vi "SingleAxis_MoveInc_MoveAbs_Home.vi"() -> ()   [LabVIEW 2016]
uses:
  Examples/Motion/EnableSingle.vi
  Examples/Motion/MoveIncSingle.vi
  Examples/Motion/WaitSingle.vi
  Examples/Motion/MoveAbsSingle.vi
  Examples/Motion/HomeSingle.vi
  Examples/Motion/DisableSingle.vi
panel:
  out "FinalPosition":string
  in  "MoveAbsPosition":dbl
  in  "MoveAbsSpeed":dbl
  in  "MoveIncDistance":dbl
  in  "MoveIncSpeed":dbl
  in  "AxisName":string
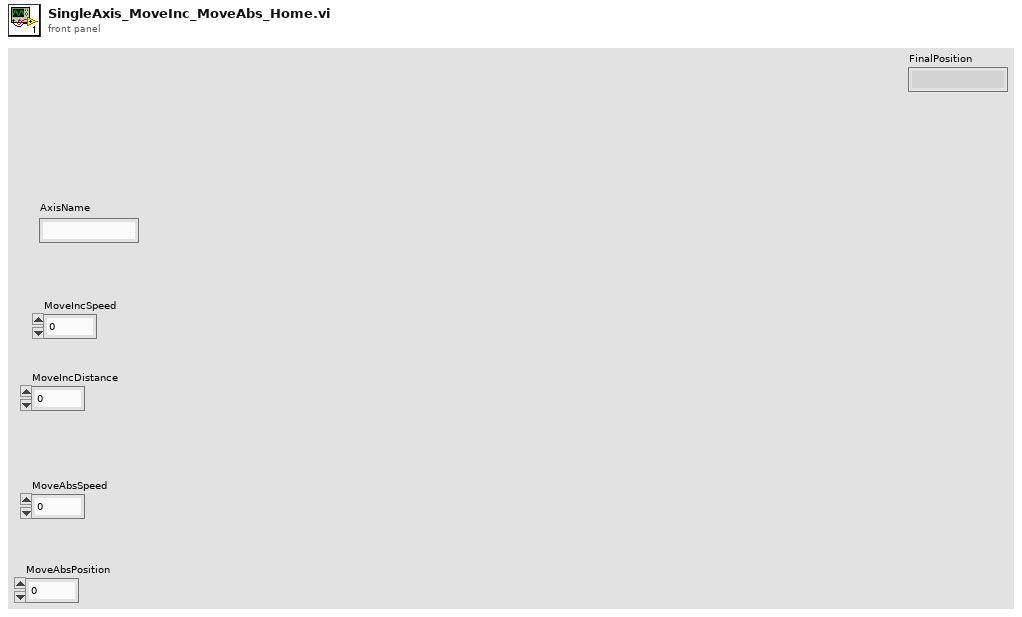
[diagram p1: front panel]
types:
  T1 = typedef "ControllerDiagPacket.ctl" = cluster{"Number of Diag Packets":i32, "Axes":T2[], "error":errorcluster}
  T2 = typedef "AxisDiagPacket.ctl" = cluster{"Axis Name":string, "Analog Input 0":dbl, "Analog Input 1":dbl, "Axis Fault (num)":i32, "Axis Fault (str)":string, "Axis Fault (bits)":cluster{"AmplifierFault":bool, "AmplifierTemperatureFault":bool, "CcwEndOfTravelLimitFault":bool, "CcwSoftwareLimitFault":bool, "CommunicationLostFault":bool, "CwEndOfTravelLimitFault":bool, "CwSoftwareLimitFault":bool, "EmergencyStopFault":bool, "EncoderFault":bool, "ExternalFault":bool, "FeedbackScalingFault":bool, "GantryMisalignFault ":bool, "HallSensorFault":bool, "InPositionTimeoutFault":bool, "MarkerSearchFault":bool, "MaxVelocityCommandFault":bool, "MissedInterruptFault":bool, "MotorTemperatureFault":bool, "None":bool, "OverCurrentFault":bool, "PositionErrorFault":bool, "PositionFeedbackFault":bool, "PowerSupplyFault":bool, "ProbeInputFault":bool, "SafeZoneFault":bool, "VelocityErrorFault":bool, "VelocityFeedbackFault":bool, "VoltageClampFault":bool}, "Axis Status (num)":i32, "Axis Status (str)":string, "Axis Status (bits)":cluster{"BacklashActive":bool, "CalibrationEnabled1D":bool, "CalibrationEnabled2D":bool, "CommandValid":bool, "DriveAbortPending":bool, "DrivePending":bool, "Enabling":bool, "GainMappingEnabled":bool, "GantryAligned":bool, "GantryRealigning":bool, "Homed":bool, "Homing":bool, "IFOVEnabled":bool, "JogGenerating":bool, "Jogging":bool, "JoystickControl":bool, "MasterSlaveControl":bool, "MotionBlocked":bool, "MotionClamped":bool, "MoveDone":bool, "None":bool, "NotVirtual":bool, "Profiling":bool, "Stability0":bool, "Stability1":bool, "TrajectoryFiltering":bool, "WaitDone":bool}, "Current Command":sgl, "Current Error":sgl, "Current Feedback":sgl, "Digital Inputs":i32, "Digital Outputs":i32, "Drive Status":i32, "Drive Status (str)":string, "Drive Status (bits)":cluster{"AccelerationPhase":bool, "AutofocusActive":bool, "BrakeOutput":bool, "CcwEndOfTravelLimitInput":bool, "CosineEncoderError":bool, "CurrentClamp":bool, "CwEndOfTravelLimitInput":bool, "DecelerationPhase":bool, "DualLoopActive":bool, "EmergencyStopInput":bool, "Enabled":bool, "EncoderClipping":bool, "GalvoCalibrationEnabled":bool, "GalvoPowerCorrection":bool, "HallAInput":bool, "HallBInput":bool, "HallCInput":bool, "HighResolutionMode":bool, "HomeLimitInput":bool, "InPosition":bool, "InPosition2":bool, "MarkerInput":bool, "MarkerLatch":bool, "MoveActive":bool, "NoMotorSupply":bool, "None":bool, "PowerLimiting":bool, "ProgrammingFlash":bool, "ProgrammingMXH":bool, "PSOHaltLatch":bool, "ServoControl":bool, "SineEncoderError":bool}, "Position Feedback Auxiliary":dbl, "Position Command":dbl, "Position Error":dbl, "Position Feedback":dbl, "Program Position Command":dbl, "Program Position Error":dbl, "Program Position Feedback":dbl, "Velocity Command":dbl, "Velocity Error":dbl, "Velocity Feedback":dbl}
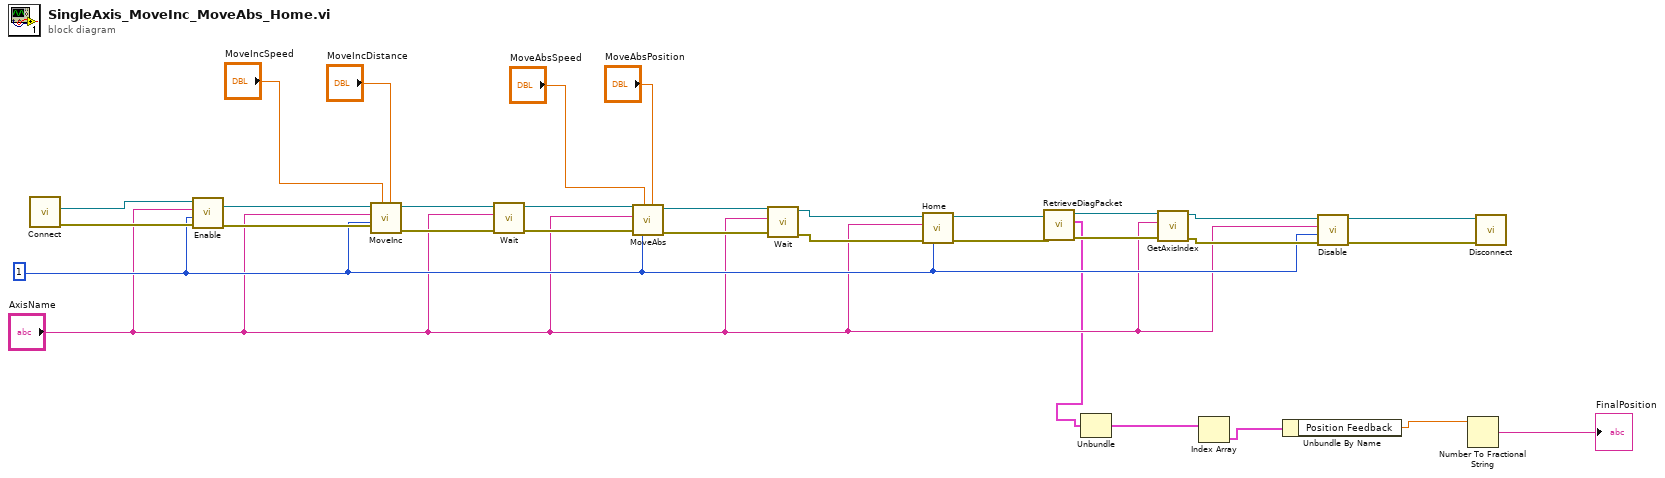
[diagram p0: block diagram]
diagram:
  w11 = 1
  n1 = call "Connect.vi"() -> ("error out"=w31:errorcluster, "controller"=w30:refnum<k24>)  [unwired: 10 in]
  n2 = call-poly "Enable.vi"("error in (no error)"=w31, "taskId"=w11, "axis name"="AxisName", "controller in"=w30) -> ("error out"=w20:errorcluster, "controller out"=w29:refnum<k24>)  [unwired: 6 in]
  n3 = call-poly "MoveInc.vi"("distance"="MoveIncDistance", "speed"="MoveIncSpeed", "error in (no error)"=w20, "taskId"=w11, "axis name"="AxisName", "controller in"=w29) -> ("error out"=w19:errorcluster, "controller out"=w28:refnum<k24>)  [unwired: 4 in]
  n4 = call-poly "Wait.vi"("error in (no error)"=w19, "axis name"="AxisName", "controller in"=w28) -> ("error out"=w18:errorcluster, "controller out"=w27:refnum<k24>)  [unwired: 6 in, 1 out]
  n5 = call-poly "MoveAbs.vi"("position"="MoveAbsPosition", "speed"="MoveAbsSpeed", "error in (no error)"=w18, "taskId"=w11, "axis name"="AxisName", "controller in"=w27) -> ("error out"=w17:errorcluster, "controller out"=w26:refnum<k24>)  [unwired: 4 in]
  n6 = call-poly "Wait.vi"("error in (no error)"=w17, "axis name"="AxisName", "controller in"=w26) -> ("error out"=w16:errorcluster, "controller out"=w25:refnum<k24>)  [unwired: 6 in, 1 out]
  n7 = call-poly "Home.vi"("error in (no error)"=w16, "taskId"=w11, "axis name"="AxisName", "controller in"=w25) -> ("error out"=w15:errorcluster, "controller out"=w24:refnum<k24>)  [unwired: 6 in]
  n8 = call "RetrieveDiagPacket.vi"("error in (no error)"=w15, "Controller In"=w24) -> ("error out"=w14:errorcluster, "ControllerDiagPacket"=w5:T1, "Controller Out"=w23:refnum<k24>)  [unwired: 7 in]
  n9 = Unbundle(w5) -> ("Axes"=w4:T2[])  [unwired: 2 out]
  n10 = call "GetAxisIndex.vi"("error in (no error)"=w14, "axis name"="AxisName", "controller in"=w23) -> ("error out"=w13:errorcluster, "controller out"=w22:refnum<k24>)  [unwired: 6 in, 1 out]
  n11 = Index Array(array=w4) -> (element=w3:T2)  [unwired: 1 in]
  n12 = Unbundle By Name(w3) -> ("Position Feedback"=w2:dbl)
  n13 = call-poly "Disable.vi"("error in (no error)"=w13, "taskId"=w11, "axis name"="AxisName", "controller in"=w22) -> ("error out"=w12:errorcluster, "controller out"=w21:refnum<k24>)  [unwired: 6 in]
  n14 = Number To Fractional String(number=w2) -> (F-format string=→"FinalPosition":string)  [unwired: 3 in]
  n15 = call "Disconnect.vi"("error in (no error)"=w12, "controller"=w21) -> ()  [unwired: 9 in, 1 out]
